vi "setPositionList.vi"(8 "error in (no error)":errorcluster, 10 "position":sgl, 11 "VGS_VolumeDescriptor+File in":refnum<class "VGS_VolumeDescriptor+File.lvclass">) -> (0 "error out":errorcluster, 2 "setPosition":bool, 3 "VGS_VolumeDescriptor+File out":refnum<class "VGS_VolumeDescriptor+File.lvclass">)   [LabVIEW 2022 SP3, in "LV_VGS.lvlib" / "VGS_VolumeDescriptor+File.lvclass"]
doc: "<B>Defines physical position of a single slice file. </B>\n\nDefines the relative physical position of a single slice file. Use this function if the file represents a single xy-slice (z-size is 1).\n\nThis function is equivalent to calling setPositionList() with a list of size 1. See setPositionList() for details. \n\n<B>bool VGS::Project::Interop::VolumeDescriptor::File::setPositionList ( List< float >^ positionList ) </B>\n\nDefines physical positions of the file's slices. \n\nDefines the relative physical position of all the slices represented by this file. Use this function to define non-equidistant slices: normally, the slice distance is determined globally by the z-component of VolumeDescriptor.Resolution, i.e. all given xy-slices are the same distance apart. If your scanned data has varying slice distances, however, you can define a kind of physical position (in mm) for each slice. These distances will then be used instead of the z-resolution value, which will be ignored.\n\n You cannot \"mix\" specifications: if you specify a position list, you must do it for all files in the VolumeDescriptor, and each file must specify as many positions as its z-size indicates! \n Optional definition. The default value is an empty list."
uses:
  VGS_VolumeDescriptor+File.lvclass
  VGS_VolumeDescriptor+File.lvclass/VGS_VolumeDescriptor+File.ctl
  C:/Users/Andrey/Documents/GitHub/LV_VGS/vgs_project.dll
  vgs_project.dll
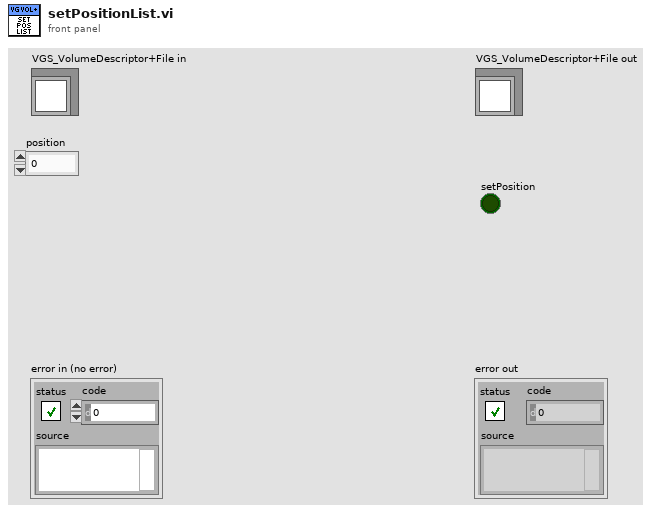
[diagram p1: front panel]
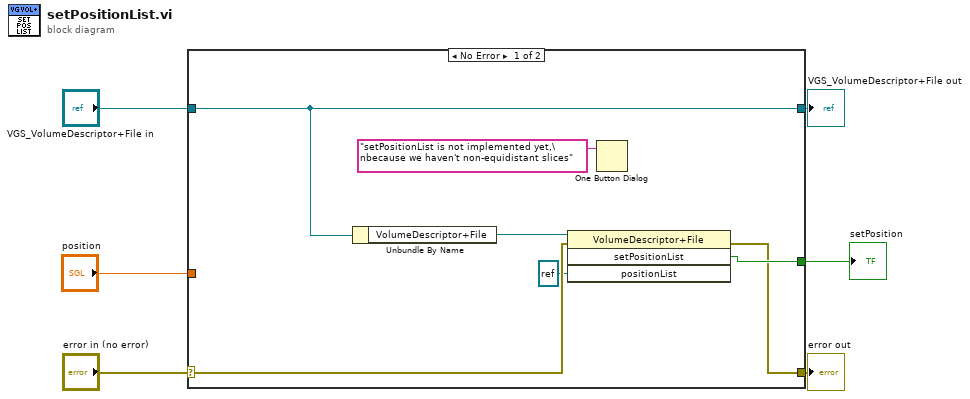
[diagram p0: block diagram]
diagram:
  n1 = case shown="No Error" "error in (no error)" {
    selector: "error in (no error)" -> [w10 w15]
    tunnel: [w9 w15] -> w5
    tunnel: [w13 w14] -> w3
    tunnel: "VGS_VolumeDescriptor+File in" -> [w13 w14]
    tunnel: "position" -> [_ _]
    tunnel: [w11 _] -> w1
    frame No Error {
      n2 = Unbundle By Name(w13) -> ("VolumeDescriptor+File"=w12:refnum<k24>)
      n3 = invoke class="VolumeDescriptor+File" method="setPositionList"(reference=w12, error in=w10, "positionList"=refnum<k24> refnum) -> (error out=w9:errorcluster, "setPositionList"=w11:bool)  [unwired: 1 in, 2 out]
      n4 = One Button Dialog(message="setPositionList is not implemented yet,\nbecause we haven't non-equidistant slices") -> ()  [unwired: 1 in, 1 out]
    }
    frame Error {
    }
  }
  "error out" <- w5
  "VGS_VolumeDescriptor+File out" <- w3
  "setPosition" <- w1
